vi "LVClass_WavefrontCorrector get Parameter Values OnlyGet.vi"(0 "WavefrontCorrector in":refnum<class "WavefrontCorrector.lvclass">, 11 "error in (no error)":errorcluster) -> (4 "WavefrontCorrector out":refnum<class "WavefrontCorrector.lvclass">, 6 "ListOfGettableValue":T1[](array[typedef]), 15 "error out":errorcluster)   [LabVIEW 2020, in "WavefrontCorrector.lvclass"]
doc: "Description:\nGet current actuators positions.\n\nParameters:\nclass corrector WavefrontCorrector object adress.\nfloat position Array containing the actuators positions.\nError error_in [in] Error\nError error_out [out] Error"
uses:
  WavefrontCorrector.lvclass
  Controls/CameraParametersSetup.ctl
  Controls/CameraParameters_Type.ctl
  WavefrontCorrector.lvclass/WavefrontCorrector.ctl
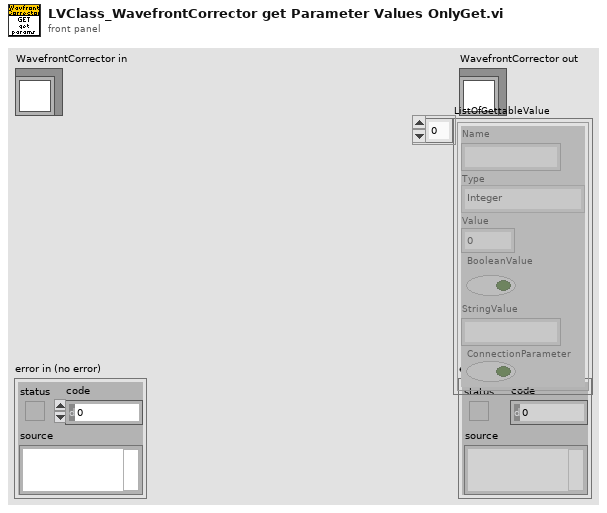
[diagram p1: front panel]
types:
  T1 = typedef "CameraParametersSetup.ctl" = cluster{"Name":string, "Type":T2, "Value":dbl, "BooleanValue":bool, "StringValue":string, "ConnectionParameter":bool}
  T2 = typedef "CameraParameters_Type.ctl" = enum16{"Integer", "Real", "String", "Boolean"}
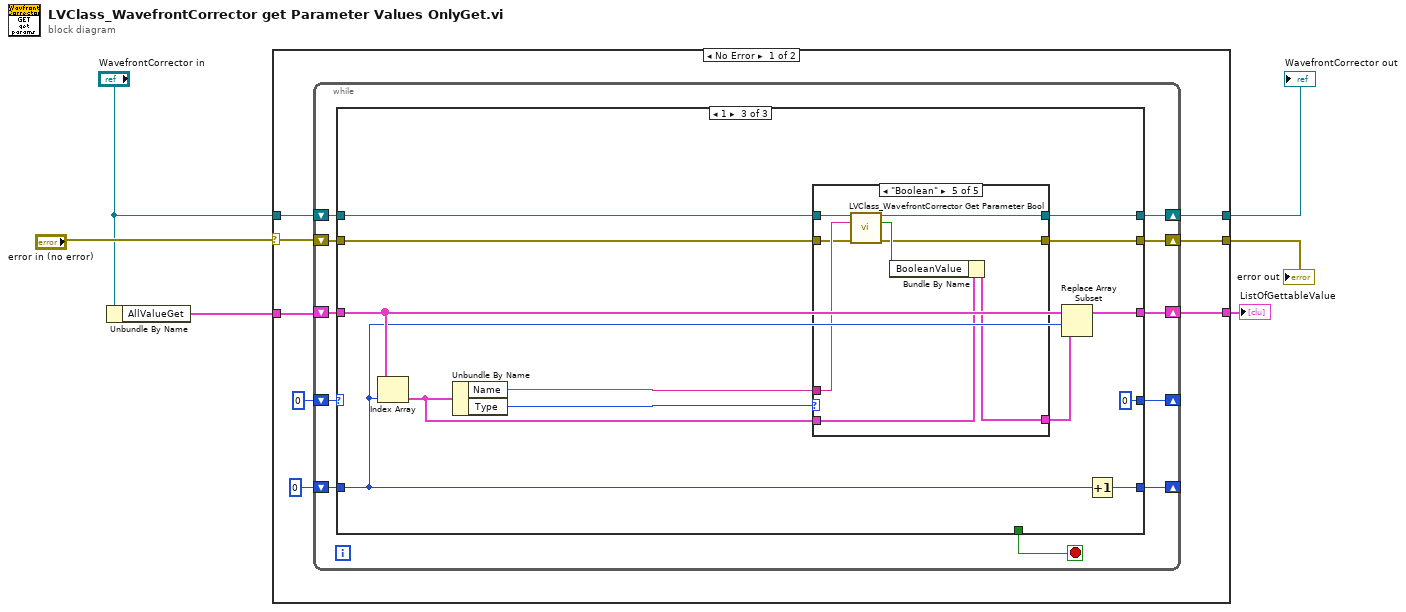
[diagram p0: block diagram]
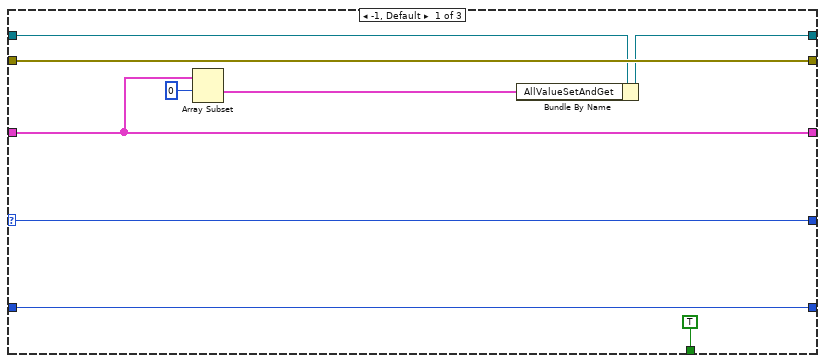
[diagram p2: hidden frame]
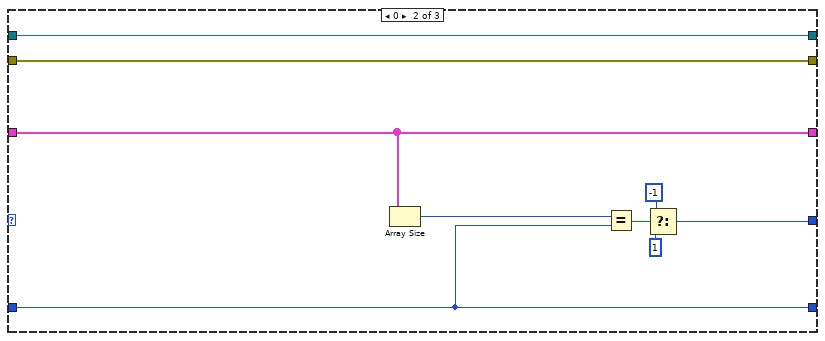
[diagram p3: hidden frame]
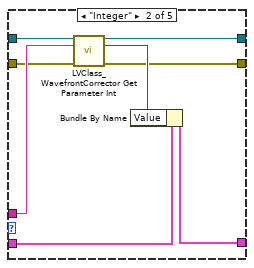
[diagram p5: hidden frame]
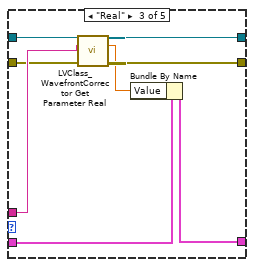
[diagram p6: hidden frame]
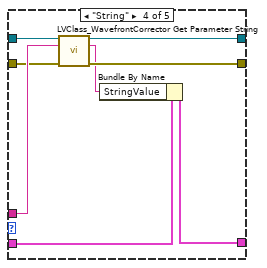
[diagram p7: hidden frame]
diagram:
  n1 = Unbundle By Name("WavefrontCorrector in") -> ("AllValueGet"=w1:T1[])
  n2 = case shown="No Error" "error in (no error)" {
    selector: "error in (no error)" -> [w10 w93]
    tunnel: [w11 w93] -> w4
    tunnel: [w12 w92] -> w6
    tunnel: "WavefrontCorrector in" -> [w14 w92]
    tunnel: [w9 _] -> w3
    tunnel: w1 -> [w7 _]
    frame No Error {
      n3 = while {
        shift-right: [w24] -> _
        shift-left: 0 -> [w23]
        shift-right: [w21] -> w11
        shift-left: w10 -> [w20]
        shift-right: [w22] -> w12
        shift-left: w14 -> [w25]
        shift-right: [w18] -> w9
        shift-left: w7 -> [w17]
        shift-right: [w15] -> _
        shift-left: 0 -> [w16]
        stop <- w19 stop-if-true
        n4 = case shown="1" w23 {
          selector: w23 -> [w31 _ _]
          tunnel: w25 -> [w27 w43 w44]
          tunnel: w20 -> [w33 w42 w45]
          tunnel: [w31 w36 0] -> w24
          tunnel: [w26 w43 w55] -> w22
          tunnel: [w33 w42 w54] -> w21
          tunnel: [TRUE _ _] -> w19
          tunnel: [w29 w41 w49] -> w18
          tunnel: w17 -> [w29 w41 w51]
          tunnel: w16 -> [w32 w39 w50]
          tunnel: [w32 w39 w53] -> w15
          frame -1, Default {
            n5 = Array Subset(array=w29, index=0) -> (w28:T1[])  [unwired: 1 in]
            n6 = Bundle By Name(cluster=w27, "AllValueSetAndGet"=w28) -> (w26:refnum<class "WavefrontCorrector.lvclass">)
          }
          frame 0 {
            n7 = Array Size(array=w41) -> (size(s)=w40:i32)
            n8 = Equal?(x=w40, y=w39) -> (x = y?=w38:bool)
            n9 = Select(t=-1, s=w38, f=1) -> (s? t:f=w36:i32)
          }
          frame 1 {
            n10 = Index Array(array=w51, index=w50) -> (element=w52:T1)
            n11 = Unbundle By Name(w52) -> ("Name"=w47:string, "Type"=w48:T2)
            n12 = case shown="\"Boolean\"" w48 {
              tunnel: w52 -> [w57 w67 w68 w76 w85]
              tunnel: [w57 w66 w69 w83 w84] -> w46
              tunnel: w47 -> [_ w65 w74 w80 w90]
              tunnel: w44 -> [w59 w64 w75 w82 w91]
              tunnel: [w59 w63 w71 w81 w88] -> w55
              tunnel: [w58 w61 w72 w78 w86] -> w54
              tunnel: w45 -> [w58 w60 w73 w79 w89]
              frame Default {
              }
              frame "Integer" {
                n13 = call "LVClass_WavefrontCorrector Get Parameter Int.vi"("WavefrontCorrector in"=w64, "parameter_name"=w65, "error in (no error)"=w60) -> ("WavefrontCorrector out"=w63:refnum<class "WavefrontCorrector.lvclass">, "value"=w62:i32, "error out"=w61:errorcluster)  [unwired: 10 in]
                n14 = Bundle By Name(cluster=w67, "Value"=w62) -> (w66:T1)
              }
              frame "Real" {
                n15 = call "LVClass_WavefrontCorrector Get Parameter Real.vi"("WavefrontCorrector in"=w75, "parameter_name"=w74, "error in (no error)"=w73) -> ("WavefrontCorrector out"=w71:refnum<class "WavefrontCorrector.lvclass">, "value"=w70:dbl, "error out"=w72:errorcluster)  [unwired: 10 in]
                n16 = Bundle By Name(cluster=w68, "Value"=w70) -> (w69:T1)
              }
              frame "String" {
                n17 = call "LVClass_WavefrontCorrector Get Parameter String.vi"("WavefrontCorrector in"=w82, "parameter_name"=w80, "error in (no error)"=w79) -> ("WavefrontCorrector out"=w81:refnum<class "WavefrontCorrector.lvclass">, "value"=w77:string, "error out"=w78:errorcluster)  [unwired: 10 in]
                n18 = Bundle By Name(cluster=w76, "StringValue"=w77) -> (w83:T1)
              }
              frame "Boolean" {
                n19 = call "LVClass_WavefrontCorrector Get Parameter Bool.vi"("WavefrontCorrector in"=w91, "parameter_name"=w90, "error in (no error)"=w89) -> ("WavefrontCorrector out"=w88:refnum<class "WavefrontCorrector.lvclass">, "value"=w87:bool, "error out"=w86:errorcluster)  [unwired: 10 in]
                n20 = Bundle By Name(cluster=w85, "BooleanValue"=w87) -> (w84:T1)
              }
            }
            n21 = Replace Array Subset(array=w51, new element=w46, index=w50) -> (w49:T1[])
            n22 = Increment(x=w50) -> (x+1=w53:i32)
          }
        }
      }
    }
    frame Error {
    }
  }
  "error out" <- w4
  "WavefrontCorrector out" <- w6
  "ListOfGettableValue" <- w3
